vi "Thermal Chamber Controller Tester.vi"() -> ()   [LabVIEW 2020]
uses:
  Thermal Chamber Controller/Private/Heater State.ctl
  Thermal Chamber Controller/Thermal Chamber Controller.lvclass
  C:/Program Files (x86)/National Instruments/LabVIEW 2020/vi.lib/Asteme/Triarc Framework/Process/Process.lvclass
  C:/Program Files (x86)/National Instruments/LabVIEW 2020/vi.lib/Asteme/Triarc Framework/View/View.lvclass
  Thermal Chamber Controller/Public/Chamber State.ctl
  <vilib>/Asteme/Triarc Framework/Process/Process.lvclass/Process.ctl
  <vilib>/Asteme/Triarc Framework/View/View.lvclass/View.ctl
  <vilib>/Asteme/Triarc Framework/Process/Public/Lifecycle/Get Lifecycle State.vi
  <vilib>/Asteme/Triarc Framework/Process/Private/SubVIs/Wait for finish.vi
  <vilib>/Asteme/Triarc Framework/Process/Protected/Messaging/Enqueue Message.vi
  <vilib>/Asteme/Triarc Framework/Process/Private/SubVIs/Set Lifecycle State.vi
  <vilib>/Asteme/Triarc Framework/View/Public/Get View VI Reference.vi
  <vilib>/Utility/error.llb/Clear Errors.vi
  <vilib>/Asteme/Triarc Framework/Process/Protected/Messaging/Request Message.vi
  <vilib>/Asteme/Triarc Framework/Process/Private/SubVIs/Enqueue Request Message.vi
  <vilib>/Asteme/Triarc Framework/View/View.lvclass
  <vilib>/Utility/error.llb/Error Cluster From Error Code.vi
  <vilib>/Asteme/Triarc Framework/Process/Private/SubVIs/Wait for Response Message.vi
  <vilib>/Asteme/Triarc Framework/Process/Process.lvclass
panel:
  out "Temperature Ramp Rate":dbl
  out "timed out?":bool
  in  "Refresh Button (sync)":bool
  in  "Refresh Button (asynchronous)":bool
  in  "Enable Heater":bool
  in  "Disable Heater":bool
  in  "Ramp Rate (deg C / second)":dbl=1.0
  in  "Temperature Set Point (deg C)":dbl=22.0
  out "Heater State":T1=enum."Heater Enabled"
  out "Actual Temperature":dbl format="%.2f"
  out "Furnace Temperature Chart":T2(graph)
  in  "Stop Module":bool
  in  "Start Module":bool
  in  "Hide Module Panel":bool
  in  "Show Module Panel":bool
  out "Status":string
  # "This VI tests the API for the Module."
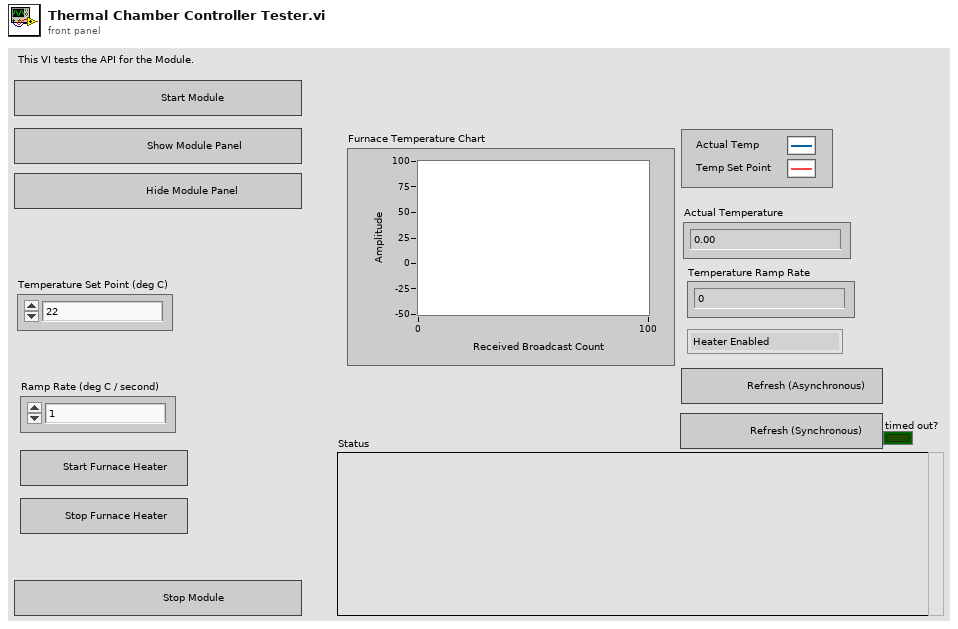
[diagram p1: front panel]
types:
  T1 = typedef "Thermal Chamber Controller.lvclass/Heater State.ctl" = enum16{"Heater Disabled", "Heater Enabled"}
  T2 = cluster{"Actual Temperature":dbl, "Required Temperature deg C":dbl}
  T3 = typedef "Thermal Chamber Controller.lvclass/Chamber State.ctl" = cluster{"Actual Temperature":dbl, "Temperature Set Point":dbl, "Temperature Ramp Rate":dbl, "Heater State":T1}
  T4 = cluster{"Actual Temperature":dbl, "Temperature Set Point":dbl}
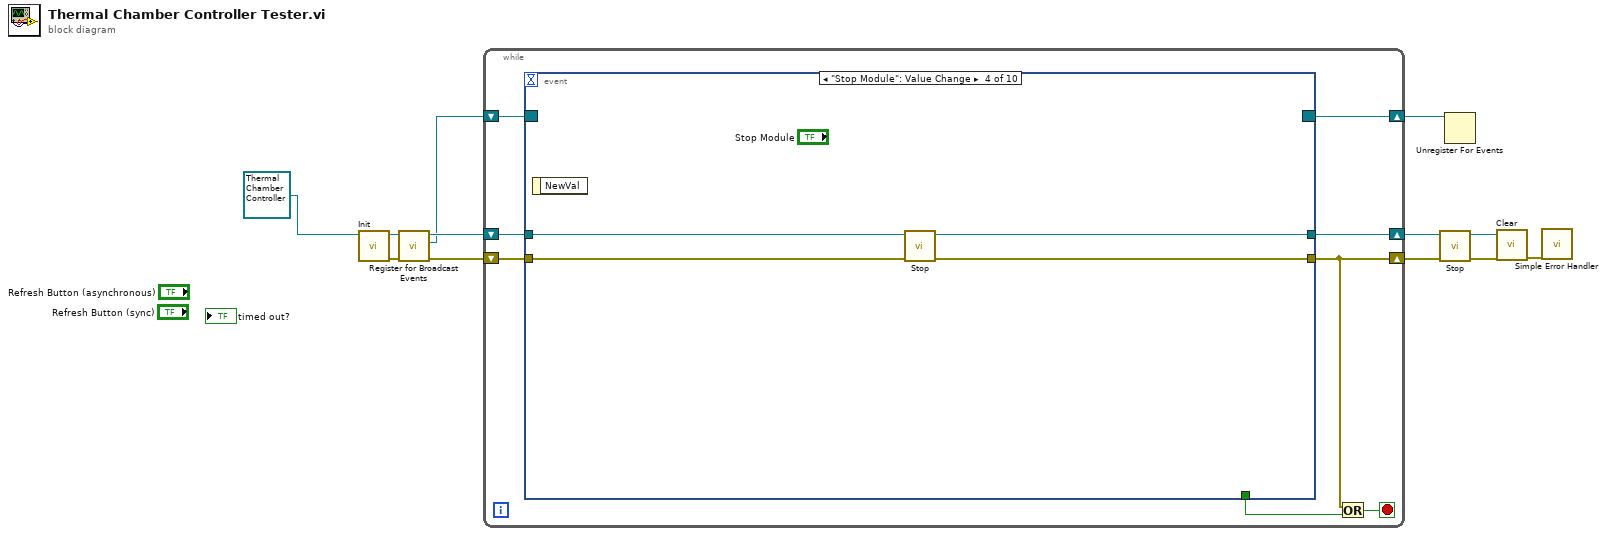
[diagram p0: block diagram]
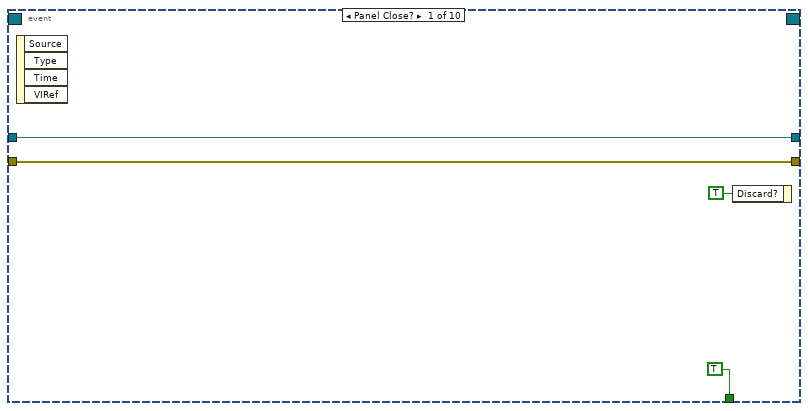
[diagram p2: hidden frame]
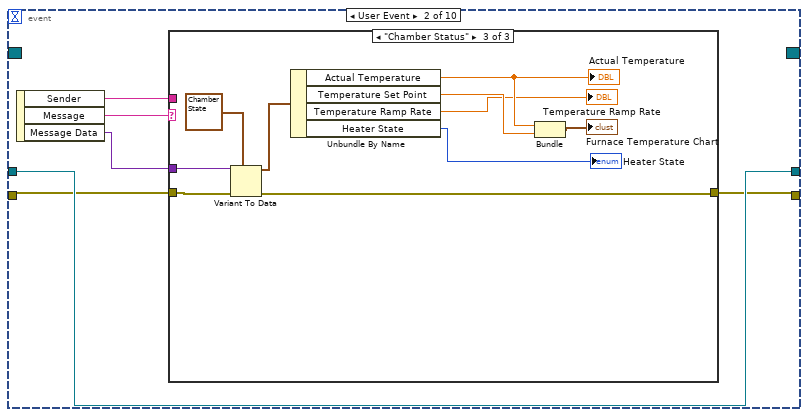
[diagram p3: hidden frame]
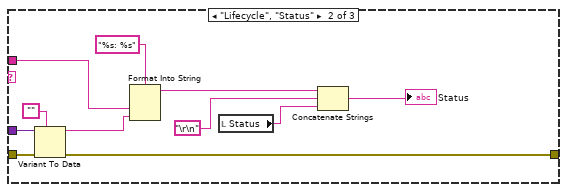
[diagram p5: hidden frame]
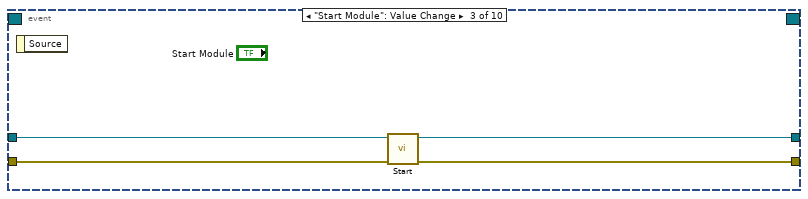
[diagram p6: hidden frame]
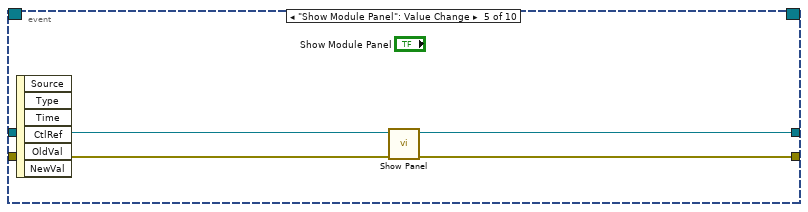
[diagram p7: hidden frame]
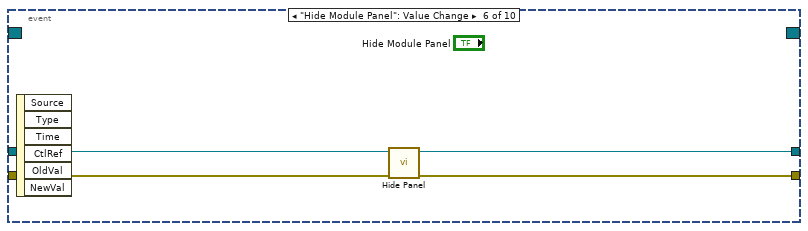
[diagram p8: hidden frame]
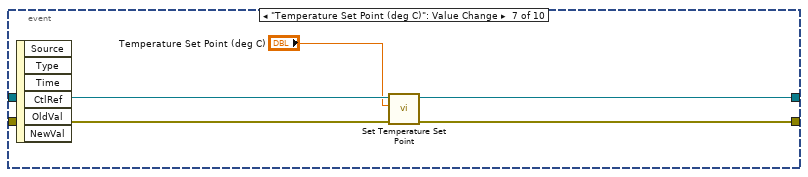
[diagram p9: hidden frame]
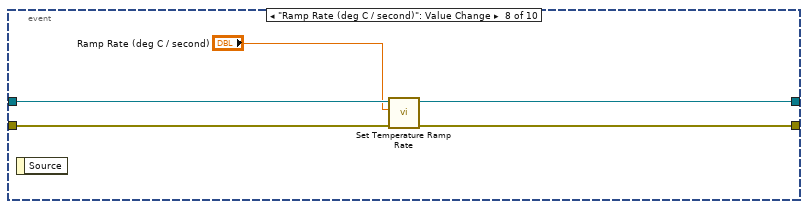
[diagram p10: hidden frame]
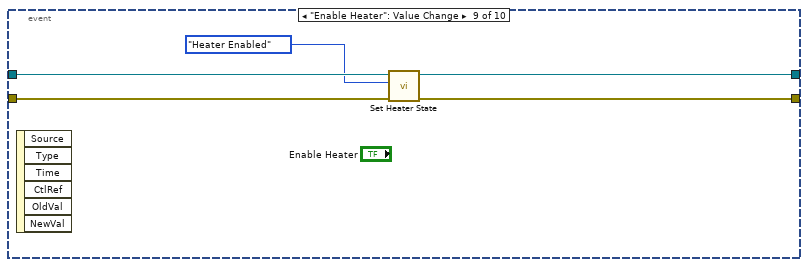
[diagram p11: hidden frame]
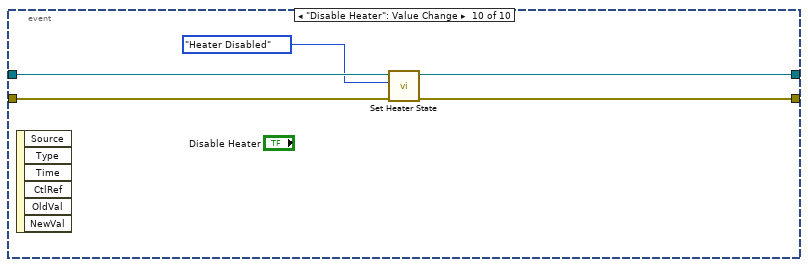
[diagram p12: hidden frame]
diagram:
  n1 = call-dynamic "Init.vi"("View In"=refnum<class "Thermal Chamber Controller.lvclass"> refnum ("Thermal Chamber Controller.lvclass")) -> ("error out"=w8:errorcluster, "View Out"=w5:refnum<class "Thermal Chamber Controller.lvclass">)  [unwired: 9 in]
  n2 = call <vilib>:"Register for Broadcast Events.vi"("error in (no error)"=w8, "Process In"=w5) -> ("error out"=w6:errorcluster, "Event Registration Refnum Out"=w3:refnum<event-registration>, "Process Out"=w4:refnum<class "Thermal Chamber Controller.lvclass">)  [unwired: 7 in]
  n3 = while {
    shift-right: [w15] -> w11
    shift-left: w6 -> [w16]
    shift-right: [w13] -> w12
    shift-left: w4 -> [w14]
    shift-right: [w18] -> w1
    shift-left: w3 -> [w19]
    stop <- w20 stop-if-true
    n4 = event shown="[3] \"Stop Module\": Value Change" {
      selector: w19 -> [_ _ _ _ _ _ _ _ _ _]
      dyn-events: [_ _ _ _ _ _ _ _ _ _] -> w18
      timeout: _ -> [_ _ _ _ _ _ _ _ _ _]
      tunnel: [TRUE _ _ _ _ _ _ _ _ _] -> w17
      tunnel: w16 -> [w23 w26 w56 w60 w64 w68 w73 w78 w83 w88]
      tunnel: [w23 w25 w55 w59 w63 w67 w72 w77 w82 w87] -> w15
      tunnel: w14 -> [w22 w30 w54 w58 w62 w66 w71 w76 w81 w86]
      tunnel: [w22 w30 w53 w57 w61 w65 w70 w75 w80 w85] -> w13
      event Panel Close? {
        n5 = event-data() -> ()  [unwired: 1 in, 4 out]
        n6 = event-data("Discard?"=TRUE) -> ()  [unwired: 1 in, 1 out]
      }
      event User Event {
        n7 = event-data() -> ("Sender"=w29:string, "Message"=w28:string, "Message Data"=w27:variant)  [unwired: 1 in]
        n8 = case shown="\"Chamber Status\"" w28 {
          tunnel: w26 -> [w31 w42 w51]
          tunnel: w27 -> [_ w41 w52]
          tunnel: w29 -> [_ w39 _]
          tunnel: [w31 w36 w50] -> w25
          frame Default {
          }
          frame "Lifecycle", "Status" {
            n9 = Variant To Data(error in=w42, type="", Variant=w41) -> (data=w38:string, error out=w36:errorcluster)
            n10 = Format Into String(format string="%s: %s", w39, w38) -> (resulting string=w34:string)  [unwired: 2 in, 1 out]
            n11 = local read "Status"() -> (w35:string)
            n12 = Concatenate Strings(w34, "\r\n", w35) -> (→"Status":string)
          }
          frame "Chamber Status" {
            n13 = Variant To Data(error in=w51, type=T3 {"Actual Temperature"=0.0, "Temperature Set Point"=0.0, "Temperature Ramp Rate"=0.0, "Heater State"=enum."Heater Enabled"} ("Chamber Status Reply Payload"), Variant=w52) -> (data=w48:T3, error out=w50:errorcluster)
            n14 = Unbundle By Name(w48) -> ("Actual Temperature"=w45:dbl, "Temperature Set Point"=w47:dbl, "Temperature Ramp Rate"=→"Temperature Ramp Rate":dbl, "Heater State"=→"Heater State":T1)
            "Actual Temperature" <- w45
            n15 = Bundle("Actual Temperature"=w45, "Temperature Set Point"=w47) -> (→"Furnace Temperature Chart":T4)  [unwired: 1 in]
          }
        }
      }
      event "Start Module": Value Change {
        n16 = event-data() -> ()  [unwired: 1 in, 1 out]
        n17 = call <vilib>:"Start.vi"("error in (no error)"=w56, "Process In"=w54) -> ("error out"=w55:errorcluster, "Process Out"=w53:refnum<class "Thermal Chamber Controller.lvclass">)  [unwired: 8 in]
      }
      event "Stop Module": Value Change {
        n18 = event-data() -> ()  [unwired: 1 in, 1 out]
        n19 = call <vilib>:"Stop.vi"("error in (no error)"=w60, "Process In"=w58) -> ("error out"=w59:errorcluster, "Process Out"=w57:refnum<class "Thermal Chamber Controller.lvclass">)  [unwired: 7 in, 1 out]
      }
      event "Show Module Panel": Value Change {
        n20 = event-data() -> ()  [unwired: 1 in, 6 out]
        n21 = call <vilib>:"Show Panel.vi"("error in (no error)"=w64, "View In"=w62) -> ("error out"=w63:errorcluster, "View Out"=w61:refnum<class "Thermal Chamber Controller.lvclass">)  [unwired: 8 in]
      }
      event "Hide Module Panel": Value Change {
        n22 = event-data() -> ()  [unwired: 1 in, 6 out]
        n23 = call <vilib>:"Hide Panel.vi"("error in (no error)"=w68, "View In"=w66) -> ("error out"=w67:errorcluster, "View Out"=w65:refnum<class "Thermal Chamber Controller.lvclass">)  [unwired: 8 in]
      }
      event "Temperature Set Point (deg C)": Value Change {
        n24 = event-data() -> ()  [unwired: 1 in, 6 out]
        n25 = call "Set Temperature Set Point.vi"("error in (no error)"=w73, "Temperature Set Point"="Temperature Set Point (deg C)", "Thermal Chamber Controller In"=w71) -> ("error out"=w72:errorcluster, "Thermal Chamber Controller Out"=w70:refnum<class "Thermal Chamber Controller.lvclass">)  [unwired: 7 in]
      }
      event "Ramp Rate (deg C / second)": Value Change {
        n26 = event-data() -> ()  [unwired: 1 in, 1 out]
        n27 = call "Set Temperature Ramp Rate.vi"("error in (no error)"=w78, "Temperature Ramp Rate [degC/s]"="Ramp Rate (deg C / second)", "Thermal Chamber Controller In"=w76) -> ("error out"=w77:errorcluster, "Thermal Chamber Controller Out"=w75:refnum<class "Thermal Chamber Controller.lvclass">)  [unwired: 7 in]
      }
      event "Enable Heater": Value Change {
        n28 = event-data() -> ()  [unwired: 1 in, 6 out]
        n29 = call "Set Heater State.vi"("error in (no error)"=w83, "Heater State"=Heater_State."Heater Enabled", "Thermal Chamber Controller In"=w81) -> ("error out"=w82:errorcluster, "Thermal Chamber Controller Out"=w80:refnum<class "Thermal Chamber Controller.lvclass">)  [unwired: 7 in]
      }
      event "Disable Heater": Value Change {
        n30 = event-data() -> ()  [unwired: 1 in, 6 out]
        n31 = call "Set Heater State.vi"("error in (no error)"=w88, "Heater State"=Heater_State."Heater Disabled", "Thermal Chamber Controller In"=w86) -> ("error out"=w87:errorcluster, "Thermal Chamber Controller Out"=w85:refnum<class "Thermal Chamber Controller.lvclass">)  [unwired: 7 in]
      }
    }
    n32 = Or(x=w15, y=w17) -> (x .or. y?=w20:bool)
  }
  n33 = call <vilib>:"Stop.vi"("error in (no error)"=w11, "Process In"=w12) -> ("error out"=w10:errorcluster, "Process Out"=w9:refnum<class "Thermal Chamber Controller.lvclass">)  [unwired: 7 in, 1 out]
  n34 = Unregister For Events(event registration refnum=w1) -> ()  [unwired: 1 in, 1 out]
  n35 = call-dynamic "Clear.vi"("error in (no error)"=w10, "View In"=w9) -> ("error out"=w2:errorcluster)  [unwired: 9 in]
  n36 = call <vilib>:"Simple Error Handler.vi"("error in (no error)"=w2) -> ()  [unwired: 4 in, 5 out]
